vi "ChangeMotorPosition.vi"() -> ()   [LabVIEW 2011]
doc: "The Basic Serial Read and Write example performs a Serial Port Read, a Serial Port Write, or a combination of these actions. The user selects the actions (read or write) on the front panel. If both are selected, the VI will write the data first, read data, and then close the VISA session that is opened to the port. This VI will wait until the specified number of bytes is received at the port or until a termination character is read.\n\nINSTRUCTIONS:\n1) Select the serial resource and configuration parameters (baud rate, data bits, parity, stop bits, flow control).\n2) Select the operations to be performed. \n3) Connect the serial port to your device. If no device is available, perform a loopback test by doing one of the following. Short pins 2 and 3 on a RS-232 cable or short pin 4 to pin 8 and pin 5 to pin 9 on a RS-485/422 cable. \n4) Run the VI to see the data read. (The \"read string\" will match the \"string to write\" if a loopback test was performed.)\n\nNote: The parameters set for the serial port must match the parameters of the connected instrument or device. In this example, the bytes to read parameter specifies the number of bytes that the serial port reads. If there were more bytes at the port than the number specified in bytes to read, those bytes would not be read. Also, if you specify to read more bytes than the number of bytes actually read, you might receive a timeout error message.\n\nOn the block diagram, the Configure Serial Port VI sets the configuration parameters. The front panel displays the controls used to configure the basic parameters, such as baud rate, data bits, and parity. Constants configure the other parameters the user probably does not need set. After the VISA Configure Serial Port VI opens the VISA session and configures the port, the VI passes the VISA resource name to other VIs that perform operations on that VISA resource. The VISA Write function sends a command to the serial device and the VISA Read function returns data based on the command. The VISA Close function then closes the reference to the serial device. It is important to close the reference; otherwise communication through with that port through protocols other than VISA might not be possible."
panel:
  out "VISA resource name out 3":refnum<visa-resource-name>
  out "error out 2":errorcluster
  in  "error out":errorcluster
  in  "VISA resource name out":refnum<visa-resource-name>
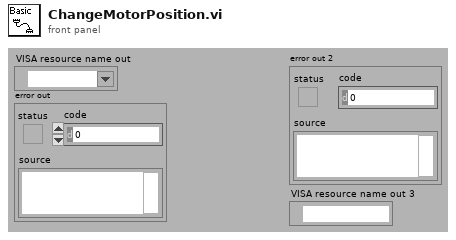
[diagram p1: front panel]
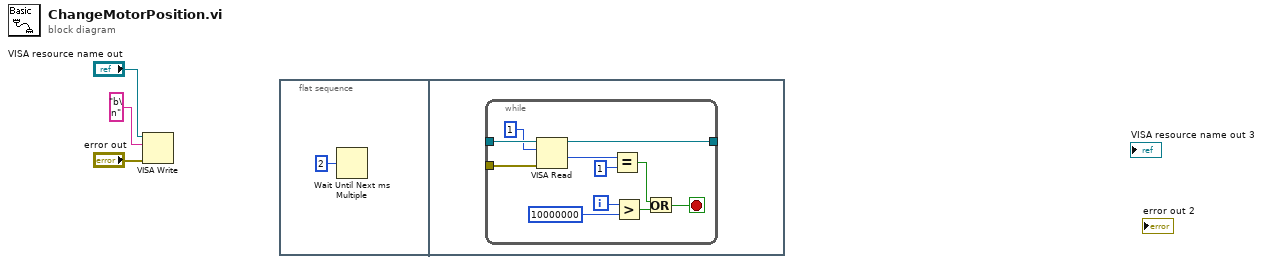
[diagram p0: block diagram]
diagram:
  n1 = VISA Write(VISA resource name="VISA resource name out", write buffer="b\n", error in (no error)="error out") -> ()  [unwired: 3 out]
  n2 = flat-sequence {
    frame #0 {
      n3 = Wait Until Next ms Multiple(millisecond multiple=u32 2) -> ()  [unwired: 1 out]
    }
    frame #1 {
      n4 = while {
        tunnel: _ -> [w15]
        tunnel: [w11] -> _
        tunnel: _ -> [w10]
        i -> [w8]
        stop <- w5 stop-if-true
        n5 = VISA Read(VISA resource name=w15, byte count=u32 1, error in (no error)=w10) -> (VISA resource name out=w11:refnum<visa-resource-name>, return count=w12:u32)  [unwired: 2 out]
        n6 = Equal?(x=w12, y=u32 1) -> (x = y?=w9:bool)
        n7 = Greater?(x=w8, y=10000000) -> (0:w7:bool)
        n8 = Or(x=w9, y=w7) -> (x .or. y?=w5:bool)
      }
    }
  }
